vi "TangoConnectSub.vi"(8 "error in (no error)":errorcluster, 11 "VISA Refnum in":refnum<visa-resource-name>="COM4") -> (0 "error out":errorcluster, 2 "function return":i32, 3 "plLSID out":i32)   [LabVIEW 2018]
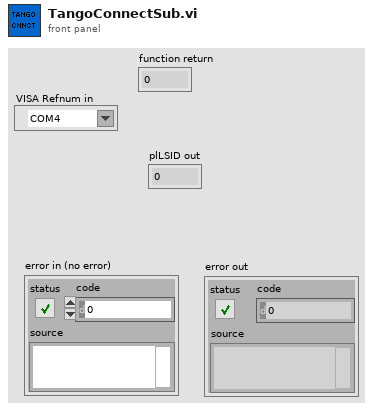
[diagram p1: front panel]
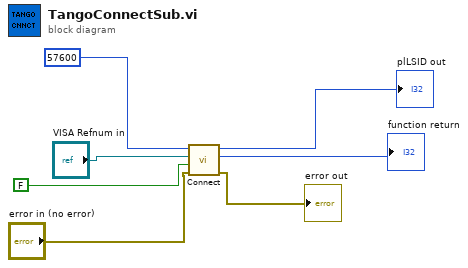
[diagram p0: block diagram]
diagram:
  n1 = call "Connect.vi"("error in (no error)"="error in (no error)", "ShProt?"=FALSE, "pcAComName"="VISA Refnum in", "lABaudRate"=57600) -> ("error out"=→"error out":errorcluster, "function return"=→"function return":i32, "plLSID out"=→"plLSID out":i32)  [unwired: 4 in]
